vi "DAQmx 9213 16ch K Thermocouple (SubVI).vi"(0 "9213 Name":tag="9213", 7 "9213 Config":T1={"Sample Rate [Hz]"=100.0, "Samples/Ch"=1, "Ch Used"=1, "Rolling Average"=1, "HI/LO Trim [%]"=1.0, "Sample Timing Engine"=2} {"Ch Used" min=1 max=16 step=1; "Sample Timing Engine" max=2; "Sample Rate [Hz]" min=0.0001 max=100.0 format="%#_6p"; "Samples/Ch" min=1 step=1; "Rolling Average" min=1 step=1; "HI/LO Trim [%]" min=1.0 max=99.0}, 11 "Error Input":errorcluster) -> (4 "Measurements":dbl[](array[numeric])=[-5.992573762181492, -5.997989953152922, -5.993374507791335, -6.01505502545452, -5.993954720178463, -5.998898340010818, -5.994243513683498, -6.001704887940654, -5.992164200481336, -5.997039559969114, -5.99175726418588, -6.014566701819755, -5.991988298982826, -5.998748692473846, -5.9949628720597365, -6.004621702529348] format="%.2f", 15 "9213 Error":errorcluster)   [LabVIEW 2012]
uses:
  <resource>/objmgr/daqmx.rc
  nilvaiu.dll
panel:
  # "DAQmx - 9213\n16ch K Thermocouple\nCreated by Blake Otting 2011\nUpdated 6-13-2013"
  # "9213 Configuration"
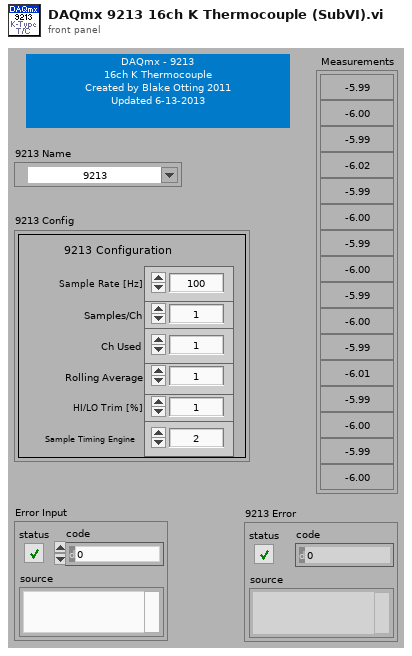
[diagram p1: front panel]
types:
  T1 = cluster{"Sample Rate [Hz]":dbl, "Samples/Ch":i32, "Ch Used":i32, "Rolling Average":i32, "HI/LO Trim [%]":dbl, "Sample Timing Engine":u32}
  T2 = cluster{"Sample Rate [Hz]":bool, "Samples/Ch":bool, "Ch Used":bool, "Rolling Average":bool, "HI/LO Trim [%]":bool, "Sample Timing Engine":bool}
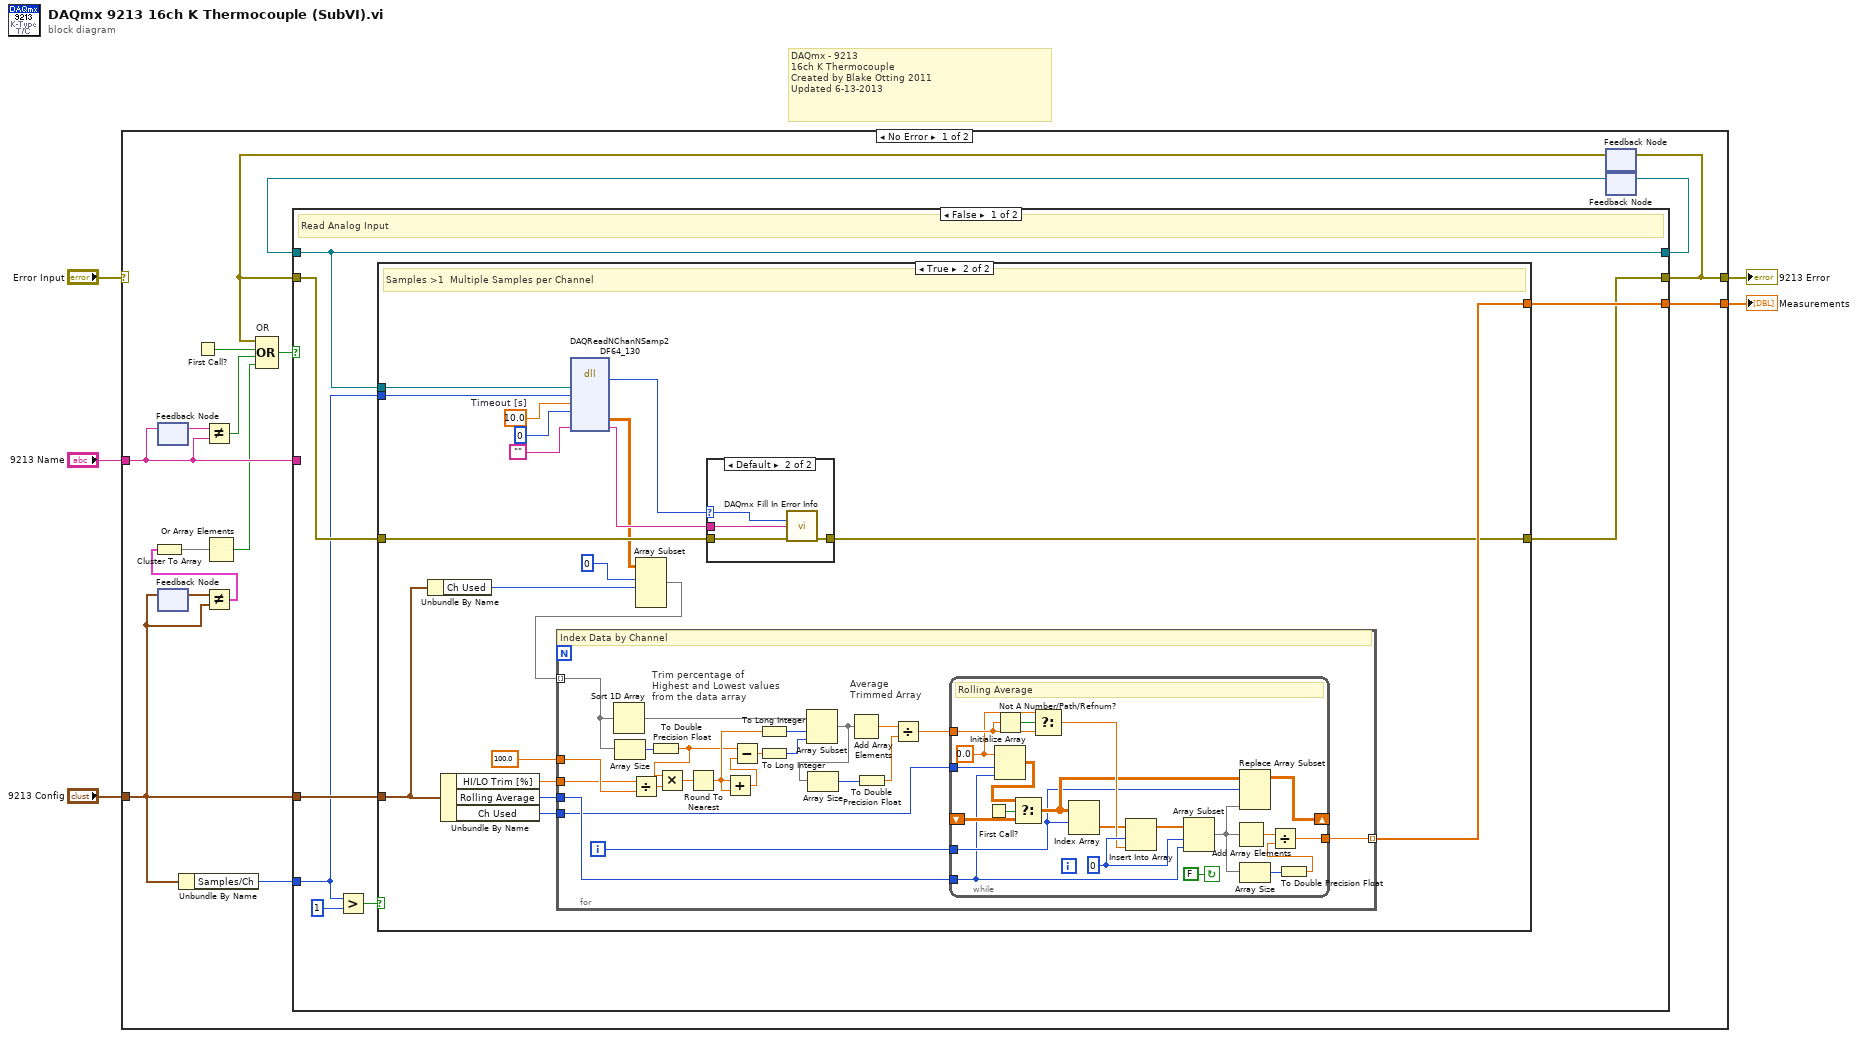
[diagram p0: block diagram]
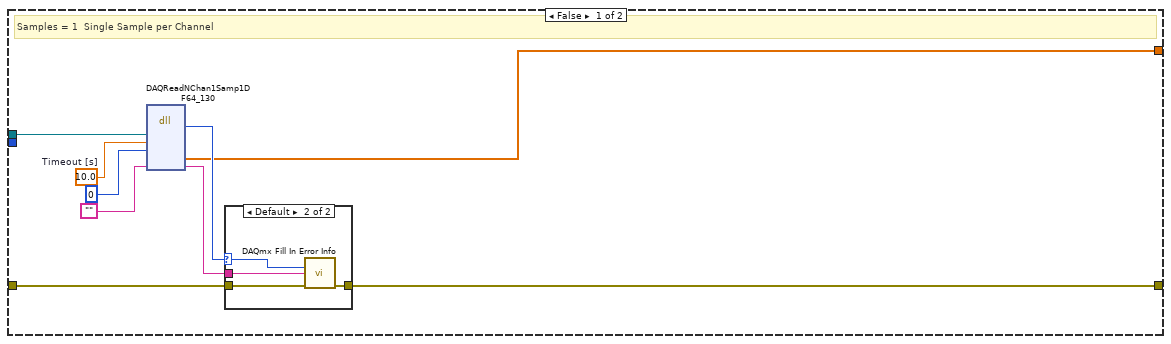
[diagram p2: hidden frame]
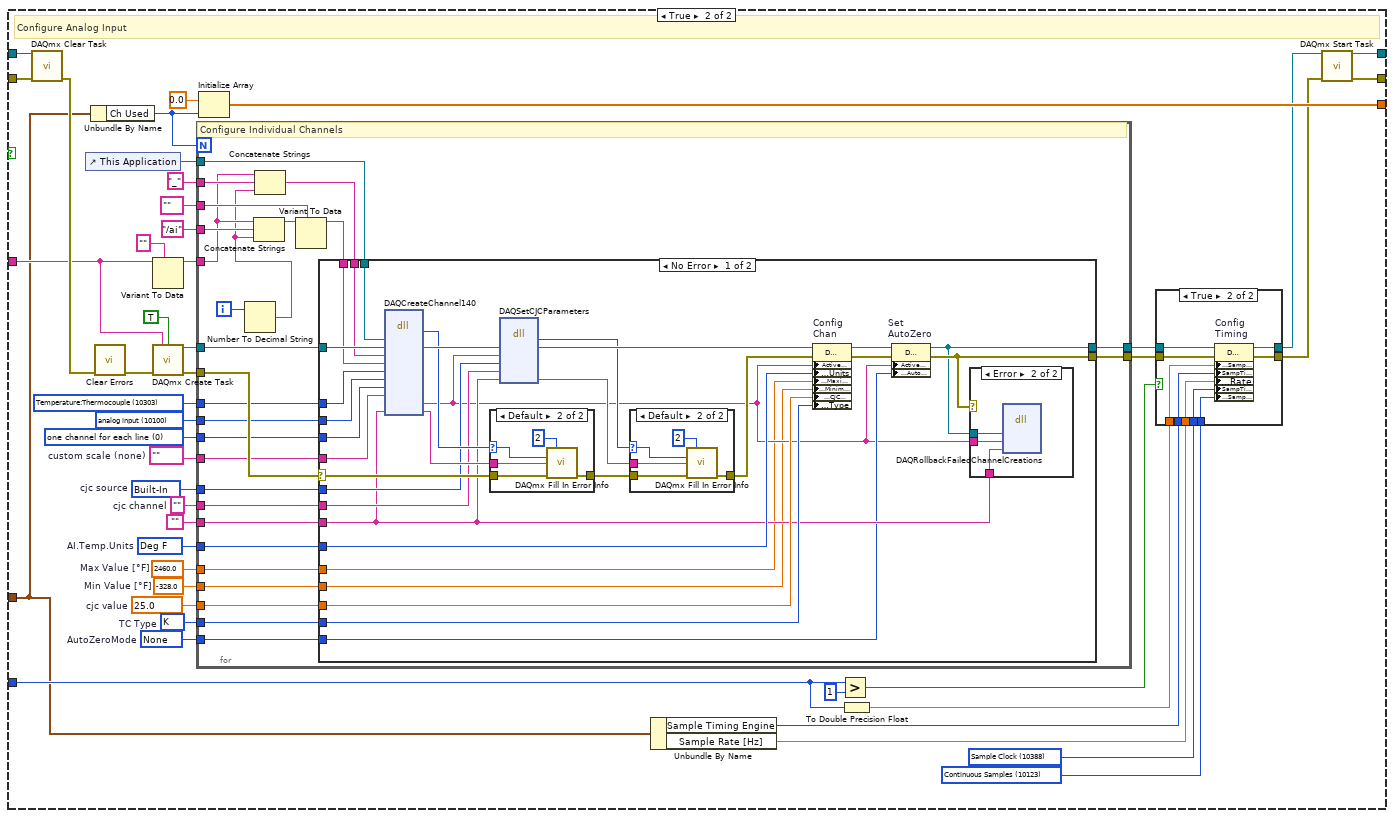
[diagram p5: hidden frame]
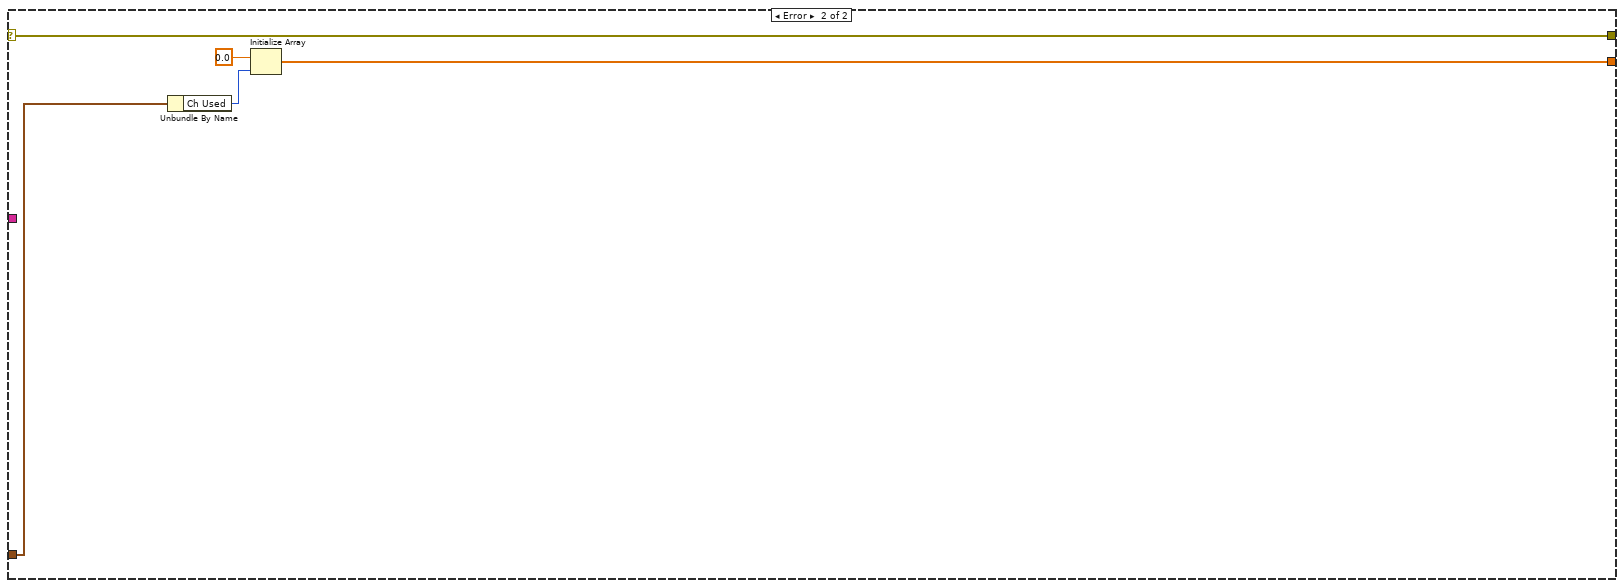
[diagram p11: hidden frame]
diagram:
  # "DAQmx - 9213\n16ch K Thermocouple\nCreated by Blake Otting 2011\nUpdated 6-13-2013"
  n1 = case shown="No Error" "Error Input" {
    selector: "Error Input" -> [_ w245]
    tunnel: [w21 w243] -> w5
    tunnel: [w15 w245] -> w3
    tunnel: "9213 Name" -> [w13 _]
    tunnel: "9213 Config" -> [w6 w242]
    frame No Error {
      n2 = feedback #1() -> (w14:tag)  [unwired: 1 in]
      n3 = feedback-in #1(w13) -> ()
      n4 = feedback #2() -> (w10:T1)  [unwired: 1 in]
      n5 = feedback-in #2(w6) -> ()
      n6 = Unbundle By Name(w6) -> ("Samples/Ch"=w11:i32)
      n7 = First Call?() -> (First Call?: T/F=w17:bool)
      n8 = Not Equal?(x=w14, y=w13) -> (x != y?=w12:bool)
      n9 = Not Equal?(x=w10, y=w6) -> (x != y?=w9:T2)
      n10 = Cluster To Array(cluster=w9) -> (array=w8:bool[])
      n11 = Or Array Elements(Boolean array=w8) -> (logical OR=w7:bool)
      n12 = feedback #3() -> (w18:errorcluster)  [unwired: 1 in]
      n13 = Compound Arithmetic op=OR "OR"(w18, w17, w12, w7) -> (w16:bool)
      n14 = feedback #4() -> (w19:refnum<k21>)  [unwired: 1 in]
      n15 = case shown="False" w16 {
        tunnel: w18 -> [w29 w151]
        tunnel: w19 -> [w28 w152]
        tunnel: w13 -> [_ w126]
        tunnel: [w28 w147] -> w20
        tunnel: [w22 w148] -> w15
        tunnel: [w26 w145] -> w21
        tunnel: w6 -> [w27 w112]
        tunnel: w11 -> [w23 w123]
        frame False {
          # "Read Analog Input"
          n16 = Greater?(x=w23, y=1) -> (0:w24:bool)
          n17 = case shown="True" w24 {
            tunnel: w23 -> [_ w53]
            tunnel: w29 -> [w32 w60]
            tunnel: w28 -> [w38 w54]
            tunnel: w27 -> [_ w46]
            tunnel: [w30 w55] -> w26
            tunnel: [w31 w48] -> w22
            frame False {
              w37 = 10.0  # Timeout [s]
              # "Samples = 1  Single Sample per Channel"
              n18 = dll-call lib="nilvaiu.dll" fn="DAQReadNChan1Samp1DF64_130" label="Read Analog Samples\nNChan 1 Samp"("taskID"=w38, "timeout"=w37, "incomingStatus"=0, "extendedErrorInfo"="") -> ("return type"=w34:i32, "data"=w30:dbl[], "extendedErrorInfo"=w33:string)  [unwired: 6 in, 3 out]
              n19 = case shown="Default" w34 {
                selector: w34 -> [_ w42]
                tunnel: [w39 w43] -> w31
                tunnel: w33 -> [_ w41]
                tunnel: w32 -> [w39 w40]
                frame 0 {
                }
                frame Default {
                  n20 = call <vilib>:"DAQmx Fill In Error Info.vi"("status code"=w42, "extended error info"=w41, "error in"=w40) -> ("error out"=w43:errorcluster)  [unwired: 1 in, 11 out]
                }
              }
            }
            frame True {
              w51 = 10.0  # Timeout [s]
              # "Samples >1  Multiple Samples per Channel"
              n21 = Unbundle By Name(w46) -> ("Ch Used"=w45:i32)
              n22 = Unbundle By Name(w46) -> ("HI/LO Trim [%]"=w47:dbl, "Rolling Average"=w57:i32, "Ch Used"=w44:i32)
              n23 = dll-call lib="nilvaiu.dll" fn="DAQReadNChanNSamp2DF64_130" label="DAQmx Read 2D\nNChan NSamp"("taskID"=w54, "samplesPerChannel"=w53, "timeout"=w51, "incomingStatus"=0, "extendedErrorInfo"="") -> (w62:i32, "data"=w49:dbl[][], "extendedErrorInfo"=w61:string)  [unwired: 7 in, 3 out]
              n24 = Array Subset(array=w49, index (row)=0, length (row)=w45) -> (w58:dbl[][])  [unwired: 2 in]
              n25 = for {
                tunnel: [w84] -> w55 mode=indexing
                tunnel: w58 -> [w63] mode=indexing
                tunnel: w47 -> [w64]
                tunnel: w57 -> [w82]
                tunnel: w44 -> [w80]
                tunnel: 100.0 -> [w65]
                i -> [w83]
                # "Average\nTrimmed Array"
                # "Trim percentage of\nHighest and Lowest values\nfrom the data array"
                # "Index Data by Channel"
                n26 = Sort 1D Array(array=w63) -> (sorted array=w72:dbl[])
                n27 = Array Size(array=w63) -> (size(s)=w78:i32)
                n28 = Divide(x=w64, y=w65) -> (x/y=w69:dbl)
                n29 = To Double Precision Float(number=w78) -> (double precision float=w70:dbl)
                n30 = Multiply(x=w70, y=w69) -> (x*y=w76:dbl)
                n31 = Round To Nearest(number=w76) -> (nearest integer value=w75:dbl)
                n32 = Add(x=w75, y=w75) -> (x+y=w71:dbl)
                n33 = Subtract(x=w70, y=w71) -> (x-y=w77:dbl)
                n34 = To Long Integer(number=w75) -> (32bit integer=w73:i32)
                n35 = To Long Integer(number=w77) -> (32bit integer=w74:i32)
                n36 = Array Subset(array=w72, index=w73, length=w74) -> (w79:dbl[])
                n37 = Array Size(array=w79) -> (size(s)=w68:i32)
                n38 = Add Array Elements(numeric array=w79) -> (sum=w67:dbl)
                n39 = To Double Precision Float(number=w68) -> (double precision float=w66:dbl)
                n40 = Divide(x=w67, y=w66) -> (x/y=w81:dbl)
                n41 = while {
                  tunnel: w81 -> [w103]
                  tunnel: w82 -> [w87]
                  shift-right: [w93] -> _
                  shift-left: _ -> [w91]
                  tunnel: [w104] -> w84
                  tunnel: w83 -> [w89]
                  tunnel: w80 -> [w86]
                  stop <- FALSE continue-if-true
                  w96 = 0.0
                  w101 = 0
                  # "Rolling Average"
                  n42 = First Call?() -> (First Call?: T/F=w98:bool)
                  n43 = Not A Number/Path/Refnum?(number/path/refnum=w103) -> (NaN/Path/Refnum?=w97:bool)
                  n44 = Initialize Array(w96, w86, w87) -> (w88:dbl[][])
                  n45 = Select(t=w88, s=w98, f=w91) -> (s? t:f=w90:dbl[][])
                  n46 = Select(t=w96, s=w97, f=w103) -> (s? t:f=w95:dbl)
                  n47 = Index Array(array=w90, index (row)=w89) -> (element=w92:dbl[])  [unwired: 1 in]
                  n48 = Insert Into Array(array=w92, index=w101, new element=w95) -> (w102:dbl[])
                  n49 = Array Subset(array=w102, index=w101, length=w87) -> (w94:dbl[])
                  n50 = Add Array Elements(numeric array=w94) -> (sum=w100:dbl)
                  n51 = Replace Array Subset(array=w90, new element=w94, index (row)=w89) -> (w93:dbl[][])  [unwired: 1 in]
                  n52 = Array Size(array=w94) -> (size(s)=w99:i32)
                  n53 = To Double Precision Float(number=w99) -> (double precision float=w85:dbl)
                  n54 = Divide(x=w100, y=w85) -> (x/y=w104:dbl)
                }
              }
              n55 = case shown="Default" w62 {
                selector: w62 -> [_ w109]
                tunnel: [w106 w110] -> w48
                tunnel: w61 -> [_ w108]
                tunnel: w60 -> [w106 w107]
                frame 0 {
                }
                frame Default {
                  n56 = call <vilib>:"DAQmx Fill In Error Info.vi"("status code"=w109, "extended error info"=w108, "error in"=w107) -> ("error out"=w110:errorcluster)  [unwired: 1 in, 11 out]
                }
              }
            }
          }
        }
        frame True {
          w113 = -328.0  # Min Value [°F]
          w114 = 2460.0  # Max Value [°F]
          w115 = 10230 items=["None"=10230, "Once"=10244, "Every Sample"=10164]  # AutoZeroMode
          w116 = 10073 items=["J"=10072, "K"=10073, "N"=10077, "R"=10082, "S"=10085, "T"=10086, "B"=10047, "E"=10055]  # TC Type
          w117 = 25.0  # cjc value
          w118 = ""  # cjc channel
          w120 = 10144 items=["Deg C"=10143, "Deg F"=10144, "Kelvins"=10325, "Deg R"=10145, "From Custom Scale"=10065]  # AI.Temp.Units
          w119 = 10200 items=["Built-In"=10200, "Constant Value"=10116, "Channel"=10113]  # cjc source
          w133 = 10123 items=["Finite Samples"=10178, "Continuous Samples"=10123, "Hardware Timed Single Point"=12522]
          w132 = 10388 items=["Sample Clock"=10388, "Handshake"=10389, "Implicit"=10451, "On Demand"=10390, "Change Detection"=12504] ("Sample Timing Type")
          w141 = tag ""  # custom scale (none)
          w142 = 10303 items=["Voltage"=10322, "Current"=10134, "More:Voltage:Custom with Excitation"=10323, "More:Current:Custom with Excitation"=10136, "Frequency"=10181, "Period"=10257, "Resistance"=10278, "Temperature:Thermocouple"=10303, "Temperature:Thermistor"=10302, "Temperature:RTD"=10301, "Temperature:Built-in Sensor"=10311, "Strain Gage"=10300] ("measurement type")
          w143 = 0 items=["one channel for each line", "one channel for all lines"] ("line grouping")
          w144 = 10100 items=["analog input"=10100, "analog output"=10102, "digital input"=10151, "digital output"=10153, "counter input"=10131, "counter output"=10132] ("channel type")
          # "Configure Analog Input"
          n57 = call <vilib>:"DAQmx Clear Task.vi"("task in"=w152, "error in"=w151) -> ("error out"=w149:errorcluster)  [unwired: 13 out]
          n58 = control-ref of="This Application"() -> (w138:refnum<vi>)
          n59 = Unbundle By Name(w112) -> ("Ch Used"=w111:i32)
          n60 = call <vilib>:"Clear Errors.vi"("error in (no error)"=w149) -> ("error out"=w150:errorcluster)  [unwired: 6 in]
          n61 = Variant To Data(type="", Variant=w126) -> (data=w125:string)  [unwired: 1 in, 1 out]
          n62 = call <vilib>:"DAQmx Create Task.vi"("new task name"=w126, "auto cleanup"=TRUE, "error in"=w150) -> ("task out"=w155:refnum<k21>, "error out"=w154:errorcluster)  [unwired: 2 in, 9 out]
          n63 = for {
            N: w111 -> [_]
            tunnel: w154 -> [w192]
            tunnel: w155 -> [w184]
            tunnel: w144 -> [w191]
            tunnel: w143 -> [w190]
            tunnel: w142 -> [w189]
            tunnel: w114 -> [w188]
            tunnel: w113 -> [w187]
            tunnel: w141 -> [w185]
            tunnel: [w183] -> w140
            tunnel: [w182] -> w139
            tunnel: w138 -> [w181]
            tunnel: "" -> [w180]
            tunnel: "/ai" -> [w179]
            tunnel: "_" -> [w178]
            tunnel: tag "" -> [w177]
            tunnel: w125 -> [w176]
            tunnel: w120 -> [w173]
            tunnel: w119 -> [w172]
            tunnel: w118 -> [w171]
            tunnel: w117 -> [w170]
            tunnel: w116 -> [w169]
            tunnel: w115 -> [w168]
            i -> [w167]
            # "Configure Individual Channels"
            n64 = Number To Decimal String(number=w167) -> (decimal integer string=w174:string)  [unwired: 1 in]
            n65 = Concatenate Strings(w176, w179, w174) -> (w193:string)
            n66 = Concatenate Strings(w176, w178, w174) -> (w186:string)
            n67 = Variant To Data(type=w177, Variant=w193) -> (data=w175:tag)  [unwired: 1 in, 1 out]
            n68 = case shown="No Error" w192 {
              selector: w192 -> [w214 w240]
              tunnel: w184 -> [w220 w239]
              tunnel: w191 -> [w212 _]
              tunnel: w190 -> [w211 _]
              tunnel: w189 -> [w213 _]
              tunnel: w188 -> [w195 _]
              tunnel: w187 -> [w194 _]
              tunnel: [w197 w239] -> w183
              tunnel: [w198 w240] -> w182
              tunnel: w186 -> [w218 _]
              tunnel: w185 -> [w210 _]
              tunnel: w175 -> [w217 _]
              tunnel: w181 -> [w219 _]
              tunnel: w180 -> [w200 _]
              tunnel: w173 -> [w201 _]
              tunnel: w172 -> [w205 _]
              tunnel: w171 -> [w204 _]
              tunnel: w170 -> [w203 _]
              tunnel: w169 -> [w202 _]
              tunnel: w168 -> [w199 _]
              frame No Error {
                n69 = dll-call lib="nilvaiu.*" fn="DAQCreateChannel140" label="Create\nAI Chan"("This Application"=w219, w220, "virtual channel name"=w218, "physical channel name"=w217, "measurement type"=w213, "channel type"=w212, "line grouping"=w211, "customScale"=w210, "extendedErrorIndo"=w200) -> (w216:i32, w223:refnum<k21>, "channel names"=w196:string, "extendedErrorIndo"=w215:string)  [unwired: 10 in, 3 out]
                n70 = case shown="Default" w216 {
                  selector: w216 -> [_ w237]
                  tunnel: [w233 w238] -> w209
                  tunnel: w215 -> [_ w235]
                  tunnel: w214 -> [w233 w234]
                  frame 0 {
                  }
                  frame Default {
                    n71 = call <vilib>:"DAQmx Fill In Error Info.vi"("depth"=2, "status code"=w237, "extended error info"=w235, "error in"=w234) -> ("error out"=w238:errorcluster)  [unwired: 1 in, 10 out]
                  }
                }
                n72 = dll-call lib="nilvaiu.*" fn="DAQSetCJCParameters" label="Set\nCJC Chan"("taskID"=w223, "activeChannel"=w196, "cjcType"=w205, "cjcChannel"=w204, "extendedErrorInfo"=w200) -> (w208:i32, "extendedErrorInfo"=w206:string)  [unwired: 6 in, 3 out]
                n73 = case shown="Default" w208 {
                  selector: w208 -> [_ w231]
                  tunnel: [w227 w232] -> w207
                  tunnel: w206 -> [_ w229]
                  tunnel: w209 -> [w227 w228]
                  frame 0 {
                  }
                  frame Default {
                    n74 = call <vilib>:"DAQmx Fill In Error Info.vi"("depth"=2, "status code"=w231, "extended error info"=w229, "error in"=w228) -> ("error out"=w232:errorcluster)  [unwired: 1 in, 10 out]
                  }
                }
                n75 = property on="Config\nChan" class="DAQmx Channel"(reference=w223, error in=w207, "Active Channels (if subset)"=w196, "Analog Input:Temperature:Units"=w201, "Analog Input:Maximum Value"=w195, "Analog Input:Minimum Value"=w194, "Analog Input:Temperature:Thermocouple:CJC Value"=w203, "Analog Input:Temperature:Thermocouple:Type"=w202) -> (reference out=w221:refnum<k21>, error out=w222:errorcluster)
                n76 = property on="Set\nAutoZero" class="DAQmx Channel"(reference=w221, error in=w222, "Active Channels (if subset)"=w196, "Analog Input:General Properties:Advanced:High Accuracy Settings:Auto Zero Mode"=w199) -> (reference out=w197:refnum<k21>, error out=w198:errorcluster)
                n77 = case shown="Error" w198 {
                  tunnel: w196 -> [_ w226]
                  tunnel: w200 -> [_ w225]
                  tunnel: w197 -> [_ w224]
                  frame No Error {
                  }
                  frame Error {
                    n78 = dll-call lib="nilvaiu.*" fn="DAQRollbackFailedChannelCreations" label="Rollback if Error"("taskID"=w224, "channelNames"=w226, "extendedErrorInfo"=w225) -> ()  [unwired: 4 in, 5 out]
                  }
                }
              }
              frame Error {
              }
            }
          }
          n79 = Initialize Array(0.0, w111) -> (w145:dbl[])
          n80 = Unbundle By Name(w112) -> ("Sample Timing Engine"=w134:u32, "Sample Rate [Hz]"=w121:dbl)
          n81 = Greater?(x=w123, y=1) -> (0:w122:bool)
          n82 = To Double Precision Float(number=w123) -> (double precision float=w131:dbl)
          n83 = case shown="True" w122 {
            tunnel: w140 -> [w157 w166]
            tunnel: w139 -> [w156 w163]
            tunnel: [w157 w165] -> w136
            tunnel: [w156 w164] -> w135
            tunnel: w134 -> [_ w161]
            tunnel: w133 -> [_ w158]
            tunnel: w132 -> [_ w159]
            tunnel: w131 -> [_ w162]
            tunnel: w121 -> [_ w160]
            frame False {
            }
            frame True {
              n84 = property on="Config\nTiming" class="DAQmx Timing"(reference=w166, error in=w163, "SampQuant.SampPerChan"=w162, "SampTimingEngine"=w161, "SampClk.Rate"=w160, "SampTimingType"=w159, "SampQuant.SampMode"=w158) -> (reference out=w165:refnum<k21>, error out=w164:errorcluster)
            }
          }
          n85 = call <vilib>:"DAQmx Start Task.vi"("task/channels in"=w136, "error in"=w135) -> ("task out"=w147:refnum<k21>, "error out"=w148:errorcluster)  [unwired: 12 in]
        }
      }
      n86 = feedback-in #3(w15) -> ()
      n87 = feedback-in #4(w20) -> ()
    }
    frame Error {
      n88 = Unbundle By Name(w242) -> ("Ch Used"=w241:i32)
      n89 = Initialize Array(0.0, w241) -> (w243:dbl[])
    }
  }
  "Measurements" <- w5
  "9213 Error" <- w3
